vi "Write roles.vi"(8 "error in (no error)":errorcluster, 10 "roles":T1, 11 "PreparePenaltyEnemyPlay in":refnum<class "PreparePenaltyEnemyPlay.lvclass">) -> (0 "error out":errorcluster, 3 "PreparePenaltyEnemyPlay out":refnum<class "PreparePenaltyEnemyPlay.lvclass">)   [LabVIEW 2023, in "PreparePenaltyEnemyPlay.lvclass"]
uses:
  PreparePenaltyEnemyPlay.lvclass
  PenaltyDefenseRole_class/PenaltyDefenseRole.lvclass
  PreparePenaltyEnemyPlay.lvclass/PreparePenaltyEnemyPlay.ctl
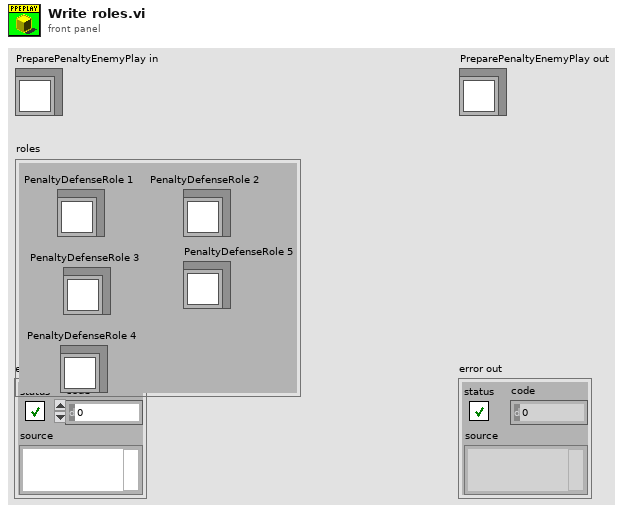
[diagram p1: front panel]
types:
  T1 = cluster{"PenaltyDefenseRole 1":refnum<class "PenaltyDefenseRole.lvclass">, "PenaltyDefenseRole 2":refnum<class "PenaltyDefenseRole.lvclass">, "PenaltyDefenseRole 3":refnum<class "PenaltyDefenseRole.lvclass">, "PenaltyDefenseRole 4":refnum<class "PenaltyDefenseRole.lvclass">, "PenaltyDefenseRole 5":refnum<class "PenaltyDefenseRole.lvclass">}
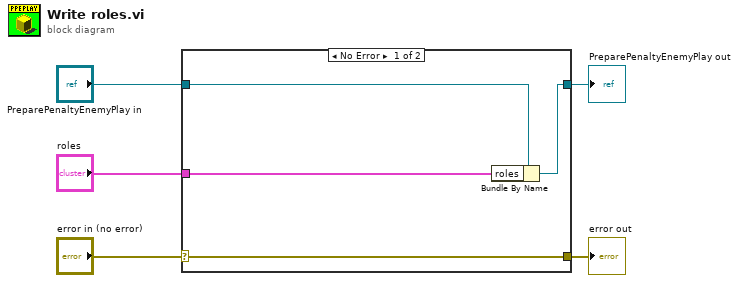
[diagram p0: block diagram]
diagram:
  n1 = case shown="No Error" "error in (no error)" {
    selector: "error in (no error)" -> [w9 w10]
    tunnel: [w9 w10] -> w4
    tunnel: [w7 w11] -> w2
    tunnel: "PreparePenaltyEnemyPlay in" -> [w8 w11]
    tunnel: "roles" -> [w6 _]
    frame No Error {
      n2 = Bundle By Name(cluster=w8, "roles"=w6) -> (w7:refnum<class "PreparePenaltyEnemyPlay.lvclass">)
    }
    frame Error {
    }
  }
  "error out" <- w4
  "PreparePenaltyEnemyPlay out" <- w2
